vi "DNA.vi"   [LabVIEW 2017]
doc: "To draw a DNA-shaped drawing on round object."
types:
  T1 = enum16{"Full", "Half", "Quarter", "Eighth", "Sixteenth"}
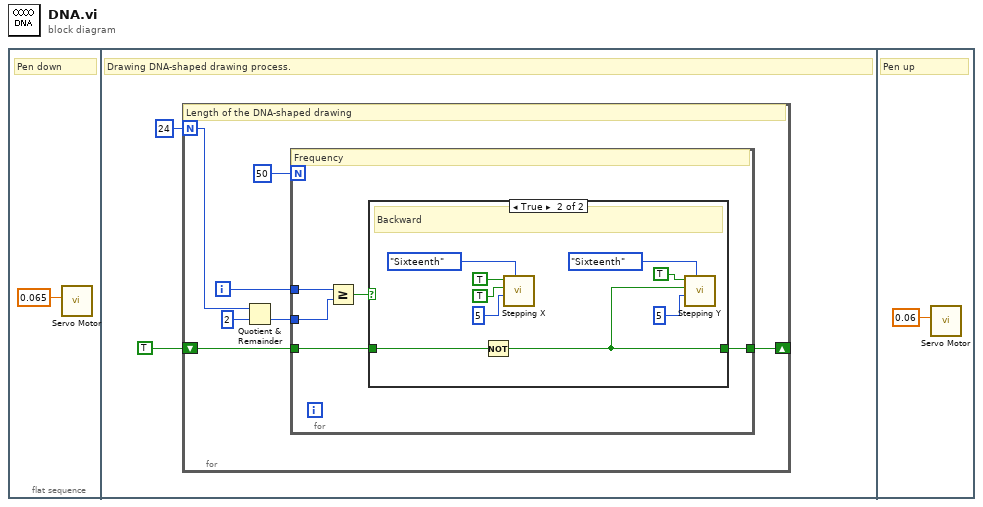
[diagram p0: block diagram]
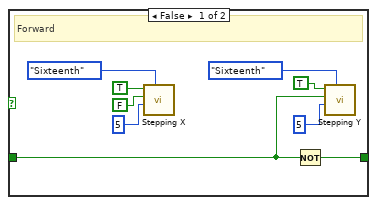
[diagram p2: hidden frame]
diagram:
  n1 = flat-sequence {
    frame #0 {
      # "Pen down"
      n2 = call "Servo Motor.vi"("Duty Cycle"=0.065) -> ()  [unwired: 10 in, 1 out]
    }
    frame #1 {
      # "Drawing DNA-shaped drawing process."
      n3 = for {
        N: 24 -> [w6]
        shift-right: [w8] -> _
        shift-left: TRUE -> [w9]
        i -> [w7]
        # "Length of the DNA-shaped drawing"
        n4 = Quotient & Remainder(x=w6, y=2) -> (floor(x/y)=w4:i32)  [unwired: 1 out]
        n5 = for {
          N: 50 -> [_]
          tunnel: w9 -> [w14]
          tunnel: [w15] -> w8
          tunnel: w7 -> [w13]
          tunnel: w4 -> [w11]
          # "Frequency"
          n6 = Greater Or Equal?(x=w13, y=w11) -> (x >= y?=w12:bool)
          n7 = case shown="True" w12 {
            tunnel: [w17 w25] -> w15
            tunnel: w14 -> [w16 w26]
            frame False {
              # "Forward"
              n8 = call "Stepping X.vi"("Microstep size"=T1."Sixteenth", "Speed"=u32 5, "Direction"=FALSE, "Enable"=TRUE) -> ()  [unwired: 7 in, 1 out]
              n9 = Not(x=w16) -> (.not. x?=w17:bool)
              n10 = call "Stepping Y.vi"("Microstep size"=T1."Sixteenth", "Speed"=u32 5, "Direction"=w16, "Enable"=TRUE) -> ()  [unwired: 7 in, 1 out]
            }
            frame True {
              # "Backward"
              n11 = Not(x=w26) -> (.not. x?=w25:bool)
              n12 = call "Stepping X.vi"("Microstep size"=T1."Sixteenth", "Speed"=u32 5, "Direction"=TRUE, "Enable"=TRUE) -> ()  [unwired: 7 in, 1 out]
              n13 = call "Stepping Y.vi"("Microstep size"=T1."Sixteenth", "Speed"=u32 5, "Direction"=w25, "Enable"=TRUE) -> ()  [unwired: 7 in, 1 out]
            }
          }
        }
      }
    }
    frame #2 {
      # "Pen up"
      n14 = call "Servo Motor.vi"("Duty Cycle"=0.06) -> ()  [unwired: 10 in, 1 out]
    }
  }
